vi "PosProcessamento_UDP_NI.vi"(1 "file path (dialog if empty)":path) -> ()   [LabVIEW 2019]
uses:
  <vilib>/Utility/file.llb/Read Delimited Spreadsheet (DBL).vi
  <vilib>/Utility/file.llb/Read Delimited Spreadsheet (string).vi
  <vilib>/Utility/file.llb/Write Delimited Spreadsheet (string).vi
panel:
  out "Arquivo":string
  out "Finalizado":bool
  out "timestamp_max":dbl format="%#_4p"
  out "j":dbl caption="Linhas da velocidade percorridas (j)"
  out "time_NI":dbl
  out "ti_UDP":dbl format="%#_9f"
  out "ti_NI":dbl format="%#_8g"
  out "NI file name":path
  out "aux":i32
  out "NI data":dbl[][](array[numeric])
  out "velocidades return":dbl[][](array[numeric])
  out "velocidades_timestamp":dbl[][](array[numeric]) format="%#_10g"
  out "velocidades_UDP":dbl[][](array[numeric])
  # "\\"
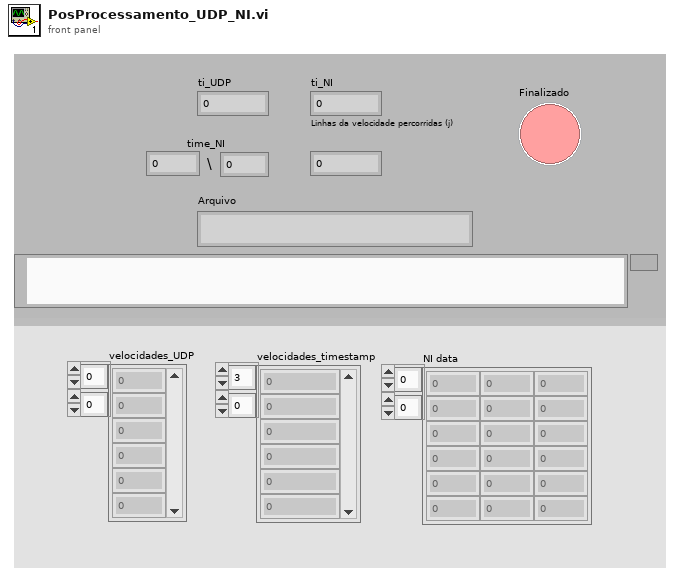
[diagram p1: front panel]
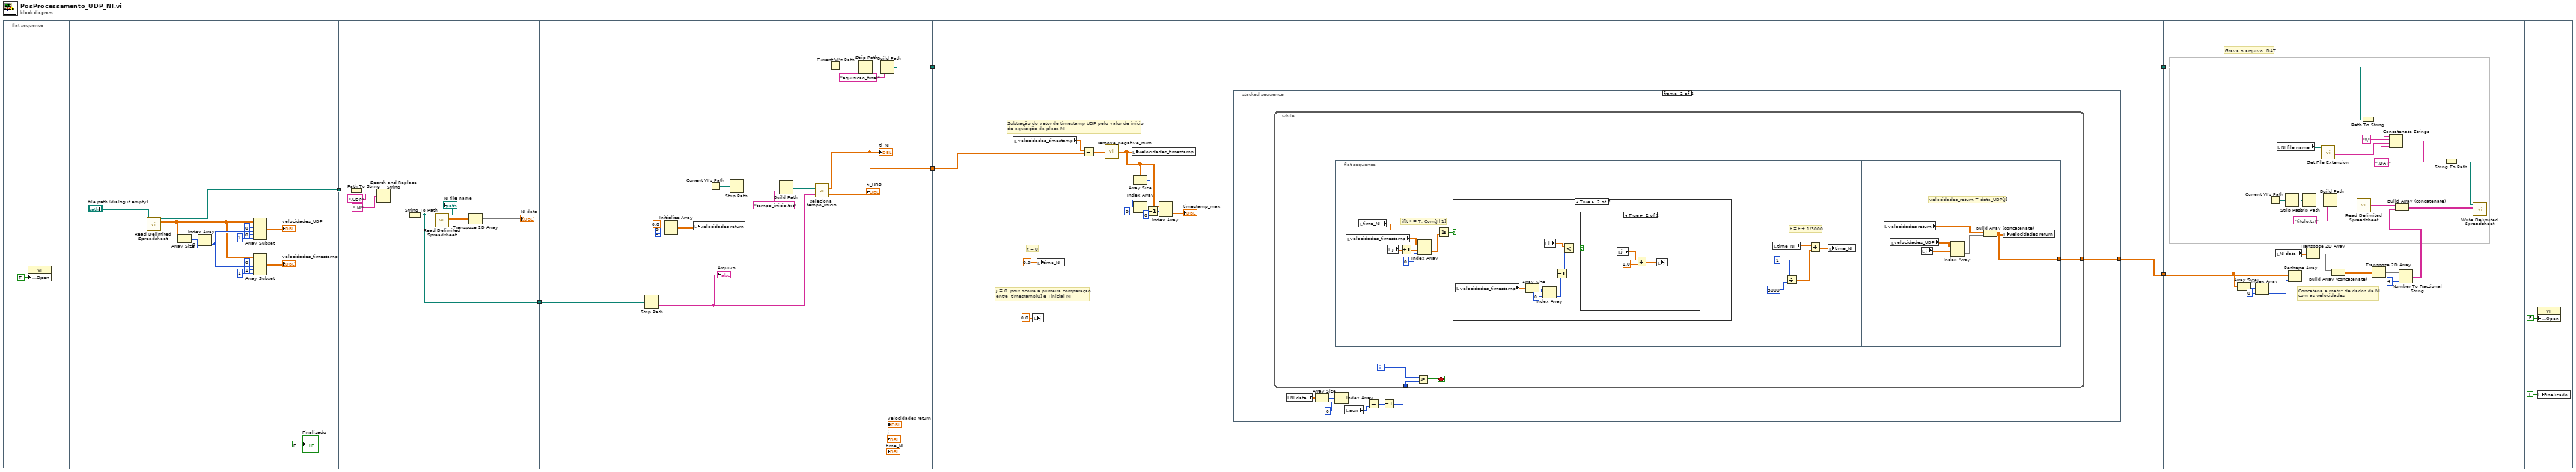
[diagram p0: block diagram]
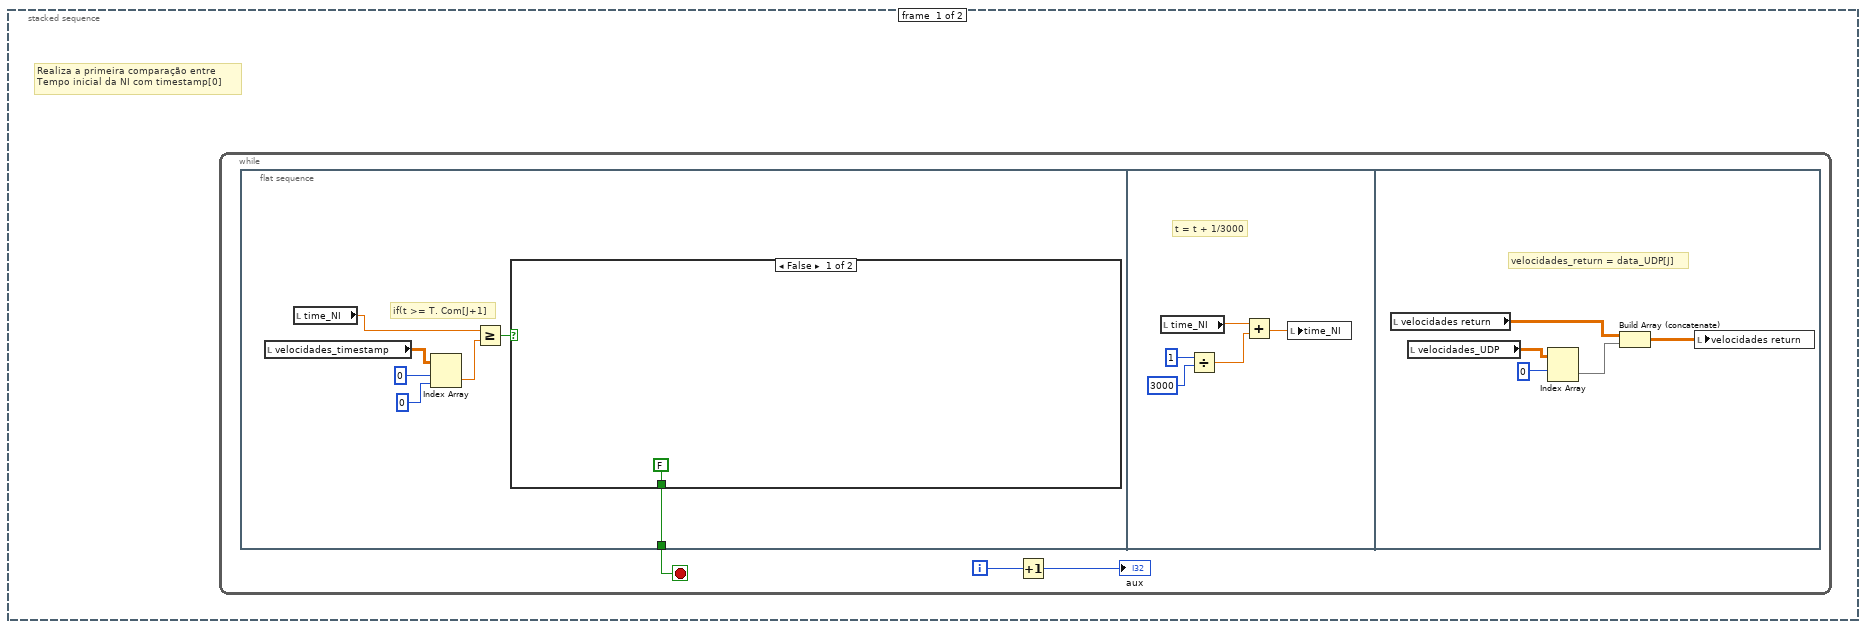
[diagram p2: hidden frame]
diagram:
  n1 = flat-sequence {
    tunnel: [w11] -> w6
    tunnel: w6 -> [w27]
    tunnel: [w23] -> w5
    tunnel: [w39] -> w4
    tunnel: w5 -> [w37]
    tunnel: [w32] -> w1
    tunnel: w4 -> [w60]
    tunnel: [w59] -> w3
    tunnel: [w48] -> w2
    tunnel: w1 -> [w48]
    tunnel: w3 -> [w132]
    tunnel: w2 -> [w122]
    frame #0 {
      n2 = property class="VI"("Front Panel.Open"=TRUE ("Front Panel Window:Open")) -> ()  [unwired: 2 in, 2 out]
    }
    frame #1 {
      n3 = call-poly <vilib>:"Read Delimited Spreadsheet.vi"("file path (dialog if empty)"="file path (dialog if empty)") -> ("new file path (Not A Path if cancelled)"=w11:path, "all rows"=w21:dbl[][])  [unwired: 9 in, 4 out]
      n4 = Array Size(array=w21) -> (size(s)=w20:i32[])
      n5 = Index Array(array=w20, index=0) -> (element=w22:i32)
      n6 = Array Subset(array=w21, index (row)=0 ("index"), length (row)=w22, index (col)=0 ("index"), length (col)=1 ("length")) -> (→"velocidades_UDP":dbl[][])
      n7 = Array Subset(array=w21, index (row)=0 ("index"), length (row)=w22, index (col)=1 ("index"), length (col)=1 ("length")) -> (→"velocidades_timestamp":dbl[][])
      "Finalizado" <- FALSE ("Finalizado")
    }
    frame #2 {
      n8 = Path To String(path=w27) -> (string=w28:string)
      n9 = Search and Replace String(input string=w28, search string=".UDP", replace string=".NI" ("replace string (\"\")")) -> (result string=w24:string)  [unwired: 5 in, 3 out]
      n10 = String To Path(string=w24) -> (path=w23:path)
      n11 = call-poly <vilib>:"Read Delimited Spreadsheet.vi"("file path (dialog if empty)"=w23) -> ("new file path (Not A Path if cancelled)"=→"NI file name":path, "all rows"=w30:dbl[][])  [unwired: 9 in, 4 out]
      n12 = Transpose 2D Array(2D array=w30) -> (transposed array=→"NI data":dbl[][])
    }
    frame #3 {
      n13 = Strip Path(path=w37) -> (name=w33:string)  [unwired: 1 out]
      "Arquivo" <- w33
      n14 = Initialize Array(0.0 ("element"), 0 ("dimension size"), 0 ("dimension size")) -> (w47:dbl[][])
      n15 = local write "velocidades return"(w47) -> ()
      n16 = Current VI's Path() -> (path=w42:path)
      n17 = Strip Path(path=w42) -> (stripped path=w41:path)  [unwired: 1 out]
      n18 = Build Path(base path=w41, name or relative path="tempo_inicio.txt") -> (appended path=w40:path)
      n19 = call "seleciona_tempo_inicio.vi"("teste"=w33, "file path (dialog if empty)"=w40) -> ("time_UDP"=→"ti_UDP":dbl, "time_NI"=w39:dbl)
      "ti_NI" <- w39
      n20 = Current VI's Path() -> (path=w36:path)
      n21 = Strip Path(path=w36) -> (stripped path=w35:path)  [unwired: 1 out]
      n22 = Build Path(base path=w35, name or relative path="aquisicao_final") -> (appended path=w32:path)
    }
    frame #4 {
      (unwired) 0 ("index")
      # "Subtração do vetor de timestamp UDP pelo valor de início\nde aquisição da placa NI"
      # "j = 0, pois ocorre a primeira comparação\nentre  timestamp[0] e Tinicial NI"
      # "t = 0"
      n23 = local read "velocidades_timestamp"() -> (w58:dbl[][])
      n24 = local write "j"(0.0 ("aux")) -> ()
      n25 = local write "time_NI"(0.0 ("time_NI")) -> ()
      n26 = Subtract(x=w58, y=w60) -> (x-y=w55:dbl[][])
      n27 = call "remove_negative_num.vi"("Array in"=w55) -> ("Array out"=w50:dbl[][])
      n28 = local write "velocidades_timestamp"(w50) -> ()
      n29 = Array Size(array=w50) -> (size(s)=w54:i32[])
      n30 = Index Array(array=w54) -> (element=w53:i32)  [unwired: 1 in]
      n31 = Decrement(x=w53) -> (x-1=w51:i32)
      n32 = Index Array(array=w50, index (row)=w51, index (col)=0 ("disabled index (col)")) -> (element=→"timestamp_max":dbl)
      n33 = stacked-sequence {
        tunnel: [_ w83] -> w59
        frame #0 {
          # "Realiza a primeira comparação entre\nTempo inicial da NI com timestamp[0]"
          n34 = while {
            i -> [w62]
            stop <- w63 stop-if-true
            n35 = flat-sequence {
              tunnel: [w64] -> w63
              frame #0 {
                # "if(t >= T. Com[J+1]"
                n36 = local read "velocidades_timestamp"() -> (w70:dbl[][])
                n37 = local read "time_NI"() -> (w66:dbl)
                n38 = Index Array(array=w70, index (row)=0 ("disabled index (row)"), index (col)=0 ("disabled index (col)")) -> (element=w69:dbl)
                n39 = Greater Or Equal?(x=w66, y=w69) -> (x >= y?=w68:bool)
                n40 = case shown="False" w68 {
                  selector: w68 -> [_ w72]
                  tunnel: [FALSE w72] -> w64
                  frame False {
                  }
                  frame True {
                  }
                }
              }
              frame #1 {
                # "t = t + 1/3000"
                n41 = local read "time_NI"() -> (w75:dbl)
                n42 = Divide(x=1, y=3000) -> (x/y=w74:dbl)
                n43 = Add(x=w75, y=w74) -> (x+y=w73:dbl)
                n44 = local write "time_NI"(w73) -> ()
              }
              frame #2 {
                # "velocidades_return = data_UDP[J]"
                n45 = local read "velocidades return"() -> (w79:dbl[][])
                n46 = local read "velocidades_UDP"() -> (w82:dbl[][])
                n47 = Index Array(array=w82, index (row)=0) -> (element=w81:dbl[])  [unwired: 1 in]
                n48 = Build Array (concatenate)(w79, w81) -> (w78:dbl[][])
                n49 = local write "velocidades return"(w78) -> ()
              }
            }
            n50 = Increment(x=w62) -> (x+1=→"aux":i32)
          }
        }
        frame #1 {
          n51 = local read "NI data"() -> (w89:dbl[][])
          n52 = Array Size(array=w89) -> (size(s)=w90:i32[])
          n53 = Index Array(array=w90, index=0) -> (element=w87:i32)
          n54 = local read "aux"() -> (w85:i32)
          n55 = Subtract(x=w87, y=w85) -> (x-y=w86:i32)
          n56 = Decrement(x=w86) -> (x-1=w84:i32)
          n57 = while {
            tunnel: w84 -> [w93]
            tunnel: [w91] -> w83
            i -> [w94]
            stop <- w92 stop-if-true
            n58 = flat-sequence {
              tunnel: [w117] -> w91
              frame #0 {
                # "if(t >= T. Com[J+1]"
                n59 = local read "velocidades_timestamp"() -> (w99:dbl[][])
                n60 = local read "time_NI"() -> (w95:dbl)
                n61 = local read "j"() -> (w100:dbl)
                n62 = Increment(x=w100) -> (x+1=w101:dbl)
                n63 = Index Array(array=w99, index (row)=w101, index (col)=0 ("disabled index (col)")) -> (element=w98:dbl)
                n64 = Greater Or Equal?(x=w95, y=w98) -> (x >= y?=w97:bool)
                n65 = case shown="True" w97 {
                  frame False {
                  }
                  frame True {
                    n66 = local read "velocidades_timestamp"() -> (w105:dbl[][])
                    n67 = Array Size(array=w105) -> (size(s)=w106:i32[])
                    n68 = Index Array(array=w106, index=0) -> (element=w103:i32)
                    n69 = local read "j"() -> (w107:dbl)
                    n70 = Decrement(x=w103) -> (x-1=w102:i32)
                    n71 = Less?(x=w107, y=w102) -> (x < y?=w108:bool)
                    n72 = case shown="True" w108 {
                      frame False {
                      }
                      frame True {
                        n73 = local read "j"() -> (w110:dbl)
                        n74 = Add(x=w110, y=1.0) -> (x+y=w111:dbl)
                        n75 = local write "j"(w111) -> ()
                      }
                    }
                  }
                }
              }
              frame #1 {
                # "t = t + 1/3000"
                n76 = local read "time_NI"() -> (w116:dbl)
                n77 = Divide(x=1, y=3000) -> (x/y=w115:dbl)
                n78 = Add(x=w116, y=w115) -> (x+y=w114:dbl)
                n79 = local write "time_NI"(w114) -> ()
              }
              frame #2 {
                # "velocidades_return = data_UDP[J]"
                n80 = local read "velocidades return"() -> (w121:dbl[][])
                n81 = local read "velocidades_UDP"() -> (w120:dbl[][])
                n82 = local read "j"() -> (w119:dbl)
                n83 = Index Array(array=w120, index (row)=w119) -> (element=w118:dbl[])  [unwired: 1 in]
                n84 = Build Array (concatenate)(w121, w118) -> (w117:dbl[][])
                n85 = local write "velocidades return"(w117) -> ()
              }
            }
            n86 = Greater Or Equal?(x=w94, y=w93) -> (x >= y?=w92:bool)
          }
        }
      }
    }
    frame #5 {
      # "Concatena a matriz de dados da NI\ncom as velocidades"
      # "Grava o arquivo .DAT"
      n87 = Array Size(array=w132) -> (size(s)=w131:i32[])
      n88 = Index Array(array=w131, index=0) -> (element=w129:i32)
      n89 = Current VI's Path() -> (path=w137:path)
      n90 = local read "NI data"() -> (w141:dbl[][])
      n91 = local read "NI file name"() -> (w128:path)
      n92 = Strip Path(path=w137) -> (stripped path=w138:path)  [unwired: 1 out]
      n93 = Reshape Array(w132, w129) -> (w133:dbl[])
      n94 = Strip Path(path=w138) -> (stripped path=w142:path)  [unwired: 1 out]
      n95 = Transpose 2D Array(2D array=w141) -> (transposed array=w135:dbl[][])
      n96 = call <vilib>:"Get File Extension.vi"("file"=w128) -> ("filename without extension"=w125:string)  [unwired: 6 in, 4 out]
      n97 = Build Path(base path=w142, name or relative path="titulo.txt") -> (appended path=w144:path)
      n98 = Build Array (concatenate)(w135, w133) -> (w134:dbl[][])
      n99 = call-poly <vilib>:"Read Delimited Spreadsheet.vi"("file path (dialog if empty)"=w144) -> ("first row"=w146:string[])  [unwired: 9 in, 5 out]
      n100 = Path To String(path=w122) -> (string=w127:string)
      n101 = Transpose 2D Array(2D array=w134) -> (transposed array=w136:dbl[][])
      n102 = Concatenate Strings(w127, "\\" ("string"), w125, ".DAT" ("string")) -> (w123:string)
      n103 = Number To Fractional String(number=w136, precision (6)=i16 4) -> (F-format string=w147:string[][])  [unwired: 2 in]
      n104 = Build Array (concatenate)(w146, w147) -> (w139:string[][])
      n105 = String To Path(string=w123) -> (path=w140:path)
      n106 = call-poly <vilib>:"Write Delimited Spreadsheet.vi"("file path (dialog if empty)"=w140, "2D data"=w139) -> ()  [unwired: 12 in, 2 out]
    }
    frame #6 {
      n107 = local write "Finalizado"(TRUE ("Finalizado")) -> ()
      n108 = property class="VI"("Front Panel.Open"=FALSE ("Front Panel Window:Open")) -> ()  [unwired: 2 in, 2 out]
    }
  }
